vi "sint64 encode.vi"(11 "sint64":i64) -> (3 "zigzag32":u64)   [LabVIEW 2013, in "protocol buffers encoder.lvlib"]
uses:
  protocol buffers encoder.lvlib
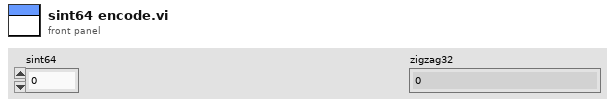
[diagram p1: front panel]
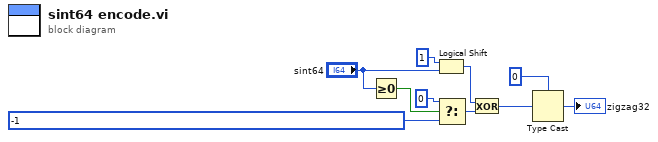
[diagram p0: block diagram]
diagram:
  n1 = Greater Or Equal To 0?(x="sint64") -> (x >= 0?=w3:bool)
  n2 = Logical Shift(y=i16 1, x="sint64") -> (x << y=w9:i64)
  n3 = Select(t=i64 0, s=w3, f=i64 -1 ("y")) -> (s? t:f=w1:i64)
  n4 = Exclusive Or(1:w1, 2:w9) -> (0:w8:i64)
  n5 = Type Cast(type=u64 0, x=w8) -> (*(type *) &x=→"zigzag32":u64)
